vi "Scan Setup.vi"(8 "error in (no error)":errorcluster, 11 "Varian Continuous in":refnum<class "Varian Continuous.lvclass">) -> (0 "error out":errorcluster, 3 "Varian Continuous out":refnum<class "Varian Continuous.lvclass">)   [LabVIEW 2009, in "Varian Continuous.lvclass"]
doc: "Configure the Instrument based on the class member fields. This step comes after the user has closed the \"Scan Setup\" window and before the actual scan -- so instruments are configured with the user's specified settings."
uses:
  Varian Continuous.lvclass
  Instruments/Varian Magnet/Varian Magnet.lvclass
  Scanner/Scanner.lvclass
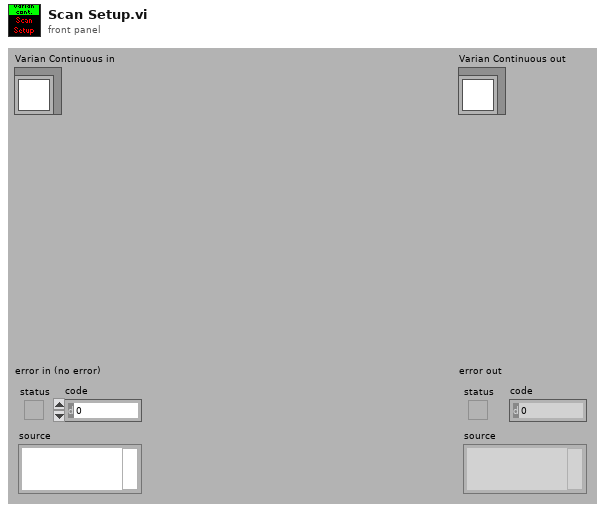
[diagram p1: front panel]
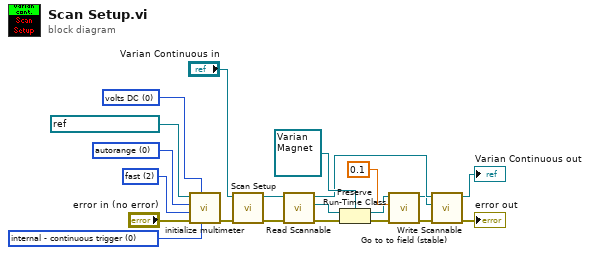
[diagram p0: block diagram]
diagram:
  w14 = u16 0 items=["volts DC", "volts AC", "2-wire k.ohms", "4-wire k.ohms", "mA DC", "mA AC"] ("function (0:volts DC)")
  w16 = u16 0 items=["autorange", "200mV, 200 ohms", "2V, 2 kohms", "20V, 20 kohms", "200V, 200 kohms", "1000Vdc, 700 Vac, 2 Mohms", "20 Mohms"] ("range (0:auto)")
  w17 = u16 2 items=["slow", "medium", "fast"] ("rate (0:slow)")
  w18 = u16 0 items=["internal - continuous trigger", "external - rear panel trigger with delay", "external - bus trigger with delay", "external - rear panel trigger", "external - bus trigger"] ("trigger mode (0:internal)")
  n1 = call "initialize multimeter.vi"("trigger mode (0:internal)"=w18, "function (0:volts DC)"=w14, "error in (no error)"="error in (no error)", "rate (0:slow)"=w17, "range (0:auto)"=w16, "VISA resource name"=refnum<visa-resource-name> "GPIB0::2::INSTR") -> ("error out"=w19:errorcluster)  [unwired: 2 in, 3 out]
  n2 = call-parent "Scan Setup.vi"("error in (no error)"=w19, "Scanner in"="Varian Continuous in") -> ("error out"=w5:errorcluster, "Scanner out"=w9:refnum<class "Varian Continuous.lvclass">)  [unwired: 8 in]
  n3 = call-dynamic "Read Scannable.vi"("error in (no error)"=w5, "Scanner.lvclass in"=w9) -> ("error out"=w11:errorcluster, "Scannable.lvclass"=w10:refnum<class "Scannable.lvclass">, "Scanner.lvclass out"=w7:refnum<class "Varian Continuous.lvclass">)  [unwired: 7 in]
  n4 = Preserve Run-Time Class(object in=w10, error in=w11, 2:refnum<class "Varian Magnet.lvclass"> refnum ("Varian Magnet.lvclass")) -> (object out=w8:refnum<class "Varian Magnet.lvclass">, error out=w4:errorcluster)
  n5 = call "Go to to field (stable).vi"("error in"=w4, "Desired field"=dbl[unit] 0.1, "varian in"=w8) -> ("error out"=w3:errorcluster, "varian out"=w2:refnum<class "Varian Magnet.lvclass">)  [unwired: 5 in, 2 out]
  n6 = call-dynamic "Write Scannable.vi"("error in (no error)"=w3, "Scannable.lvclass"=w2, "Scanner.lvclass in"=w7) -> ("error out"=→"error out":errorcluster, "Scanner.lvclass out"=→"Varian Continuous out":refnum<class "Varian Continuous.lvclass">)  [unwired: 7 in]
